vi "SPD.Config Read Test03a DTvsInsens.vi"(8 "Error In":errorcluster, 11 "SPD.Stand Ctrl in":T2={"spdDeviceSession"={"spdRef"=0, "connected"=FALSE, "spdName"="", "specification"={"diod case"=enum."default", "type"=enum."Unknown", "frequency"=enum."Unknown"}, "hidSPD.Controller"={"TSet"=0.0, "HV_bias"=0.0, "DDS_stb_code"=0}, "hidSPD.Sturtup Values"={"TSet"=0.0, "HV_bias"=0.0, "DDS_stb_code"=0}}, "DevBSession"={"DevBRef"="", "connected"=FALSE}, "FreqCSession"={"FreqCRef"="", "timeout"=0.0, "Gate"=0.0, "connected"=FALSE}, "8164BSession"={"Connection ID"=refnum, "Connected"=FALSE, "Info"="", "Slots Info"=[]}, "LeCroySession"={"LeCroySession"="", "connected"=FALSE}, "Events"={"DCRTest"=refnum, "Stop"=refnum}, "configFile"={"configFile ref"=refnum, "configFile path"=path "", "equipmentFile ref"=refnum}, "SPD.Meas Grid"={"DateTime"="", "DT"=[], "Insensitivity"=[], "Temprature"=[], "Stb_code"=[], "HV_Bias"=[]}, "SPD.Queues"={"state queue"=refnum}, "Console"=refnum} {"spdDeviceSession"."hidSPD.Sturtup Values"."HV_bias" format="%#_6p, V"; "spdDeviceSession"."hidSPD.Sturtup Values"."TSet" format="%#_6p, DegC"; "spdDeviceSession"."hidSPD.Controller"."HV_bias" format="%#_6p, V"; "spdDeviceSession"."hidSPD.Controller"."TSet" format="%#_6p, DegC"}) -> (0 "Error Out":errorcluster, 2 "DTvsInsens Params":T1, 3 "SPD.Stand Ctrl out":T2={"spdDeviceSession"={"spdRef"=0, "connected"=FALSE, "spdName"="", "specification"={"diod case"=enum."default", "type"=enum."Unknown", "frequency"=enum."Unknown"}, "hidSPD.Controller"={"TSet"=0.0, "HV_bias"=0.0, "DDS_stb_code"=0}, "hidSPD.Sturtup Values"={"TSet"=0.0, "HV_bias"=0.0, "DDS_stb_code"=0}}, "DevBSession"={"DevBRef"="", "connected"=FALSE}, "FreqCSession"={"FreqCRef"="", "timeout"=0.0, "Gate"=0.0, "connected"=FALSE}, "8164BSession"={"Connection ID"=refnum, "Connected"=FALSE, "Info"="", "Slots Info"=[]}, "LeCroySession"={"LeCroySession"="", "connected"=FALSE}, "Events"={"DCRTest"=refnum, "Stop"=refnum}, "configFile"={"configFile ref"=refnum, "configFile path"=path "", "equipmentFile ref"=refnum}, "SPD.Meas Grid"={"DateTime"="", "DT"=[], "Insensitivity"=[], "Temprature"=[], "Stb_code"=[], "HV_Bias"=[]}, "SPD.Queues"={"state queue"=refnum}, "Console"=refnum} {"spdDeviceSession"."hidSPD.Sturtup Values"."HV_bias" format="%#_6p, V"; "spdDeviceSession"."hidSPD.Sturtup Values"."TSet" format="%#_6p, DegC"; "spdDeviceSession"."hidSPD.Controller"."HV_bias" format="%#_6p, V"; "spdDeviceSession"."hidSPD.Controller"."TSet" format="%#_6p, DegC"})   [LabVIEW 2018]
uses:
  typedefs/SPD.Stand Ctrl.ctl
  Instruments/SPD HID Interface/hidSPDLibForLabView/LibVIs/hidSPD Controls/hidSPD Device Session.ctl
  Instruments/SPD HID Interface/hidSPDLibForLabView/LibVIs/hidSPD Controls/hidSPD.SPD specification.ctl
  Instruments/SPD HID Interface/hidSPDLibForLabView/LibVIs/hidSPD Controls/hidSPD SPD Diod Case.ctl
  Instruments/SPD HID Interface/hidSPDLibForLabView/LibVIs/hidSPD Controls/hidSPD SPD Type.ctl
  Instruments/SPD HID Interface/hidSPDLibForLabView/LibVIs/hidSPD Controls/hidSPD.STB Frequency.ctl
  Instruments/SPD HID Interface/hidSPDLibForLabView/LibVIs/hidSPD Controls/hidSPD Controller.ctl
  Instruments/KC705 DevBoard/typedefs/DevB.Session.ctl
  Instruments/KeySight 53230A/typedefs/FreqC.Session.ctl
  Instruments/KeySight 8164B/KeySight 8164B LAN InstrLib/typedefs/KeySight 8164B control.ctl
  Instruments/LeCroy SDA830/typedefs/LeCroy.Session.ctl
  typedefs/SPD.Events.ctl
  SPD.Config File ctrl.ctl
  <vilib>/Utility/config.llb/Config Data RefNum.ctl
  typedefs/SPD.Meas Grid.ctl
  typedefs/SPD.Queues.ctl
  typedefs/SPD.Stand state.ctl
  SPD Measurements/DT&Insensitivity/typedefs/SPD.DT&Insens Test Params.ctl
  <vilib>/Utility/config.llb/Read Key (I32).vi
  <vilib>/Utility/config.llb/Read Key (Double).vi
  <vilib>/Utility/config.llb/Read Key (String).vi
  <vilib>/Utility/config.llb/NI_LVConfig.lvlib
  Instruments/KeySight 8164B/KeySight 8164B LAN InstrLib.lvlib
  Instruments/SPD HID Interface/hidSPDLibForLabView/hidSPDLibForLabView.lvlib
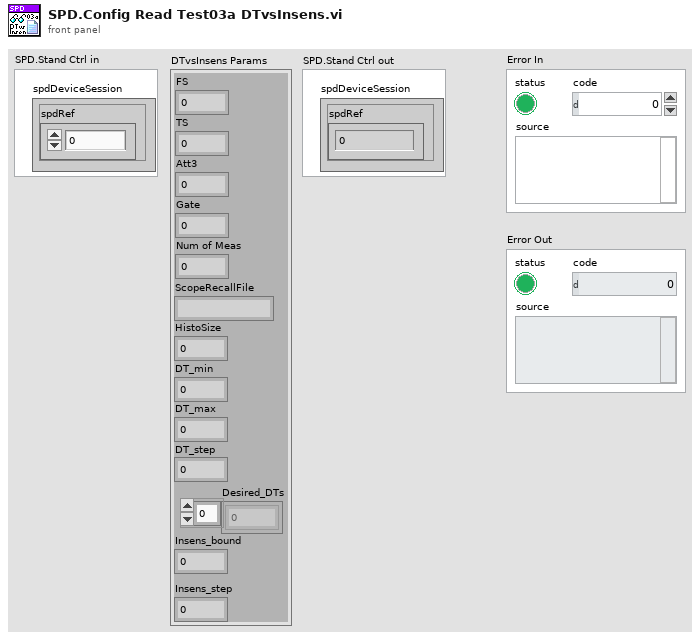
[diagram p1: front panel]
types:
  T1 = typedef "SPD.DT&Insens Test Params.ctl" = cluster{"FS":i32, "TS":i32, "Att3":dbl, "Gate":dbl, "Num of Meas":i32, "ScopeRecallFile":string, "HistoSize":i32, "DT_min":u16, "DT_max":u16, "DT_step":u16, "Desired_DTs":dbl[], "Insens_bound":u16, "Insens_step":u16}
  T2 = typedef "SPD.Stand Ctrl.ctl" = cluster{"spdDeviceSession":T3, "DevBSession":T9, "FreqCSession":T10, "8164BSession":T11, "LeCroySession":T12, "Events":T13, "configFile":T14, "SPD.Meas Grid":T16, "SPD.Queues":T17, "Console":refnum<vi>}
  T3 = typedef "hidSPDLibForLabView.lvlib/hidSPD Device Session.ctl" = cluster{"spdRef":u64, "connected":bool, "spdName":string, "specification":T4, "hidSPD.Controller":T8, "hidSPD.Sturtup Values":T8}
  T4 = typedef "hidSPDLibForLabView.lvlib/hidSPD.SPD specification.ctl" = cluster{"diod case":T5, "type":T6, "frequency":T7}
  T5 = typedef "hidSPDLibForLabView.lvlib/hidSPD SPD Diod Case.ctl" = enum16{"Unknown", "default", "butterfly"}
  T6 = typedef "hidSPDLibForLabView.lvlib/hidSPD SPD Type.ctl" = enum16{"Unknown", "Free Run", "Gate"}
  T7 = typedef "hidSPDLibForLabView.lvlib/hidSPD.STB Frequency.ctl" = enum16{"Unknown", "312", "1250"}
  T8 = typedef "hidSPDLibForLabView.lvlib/hidSPD Controller.ctl" = cluster{"TSet":sgl, "HV_bias":sgl, "DDS_stb_code":u16}
  T9 = typedef "DevB.Session.ctl" = cluster{"DevBRef":refnum<visa-resource-name>, "connected":bool}
  T10 = typedef "FreqC.Session.ctl" = cluster{"FreqCRef":refnum<visa-resource-name>, "timeout":dbl, "Gate":dbl, "connected":bool}
  T11 = typedef "KeySight 8164B LAN InstrLib.lvlib/KeySight 8164B control.ctl" = cluster{"Connection ID":refnum<k5>, "Connected":bool, "Info":string, "Slots Info":string[]}
  T12 = typedef "LeCroy.Session.ctl" = cluster{"LeCroySession":refnum<visa-resource-name>, "connected":bool}
  T13 = typedef "SPD.Events.ctl" = cluster{"DCRTest":refnum<user-event>, "Stop":refnum<user-event>}
  T14 = typedef "SPD.Config File ctrl.ctl" = cluster{"configFile ref":T15, "configFile path":path, "equipmentFile ref":T15}
  T15 = typedef "NI_LVConfig.lvlib/Config Data RefNum.ctl" = refnum<k1>
  T16 = typedef "SPD.Meas Grid.ctl" = cluster{"DateTime":string, "DT":dbl[], "Insensitivity":dbl[], "Temprature":dbl[], "Stb_code":dbl[], "HV_Bias":dbl[][][][]}
  T17 = typedef "SPD.Queues.ctl" = cluster{"state queue":refnum<queue>}
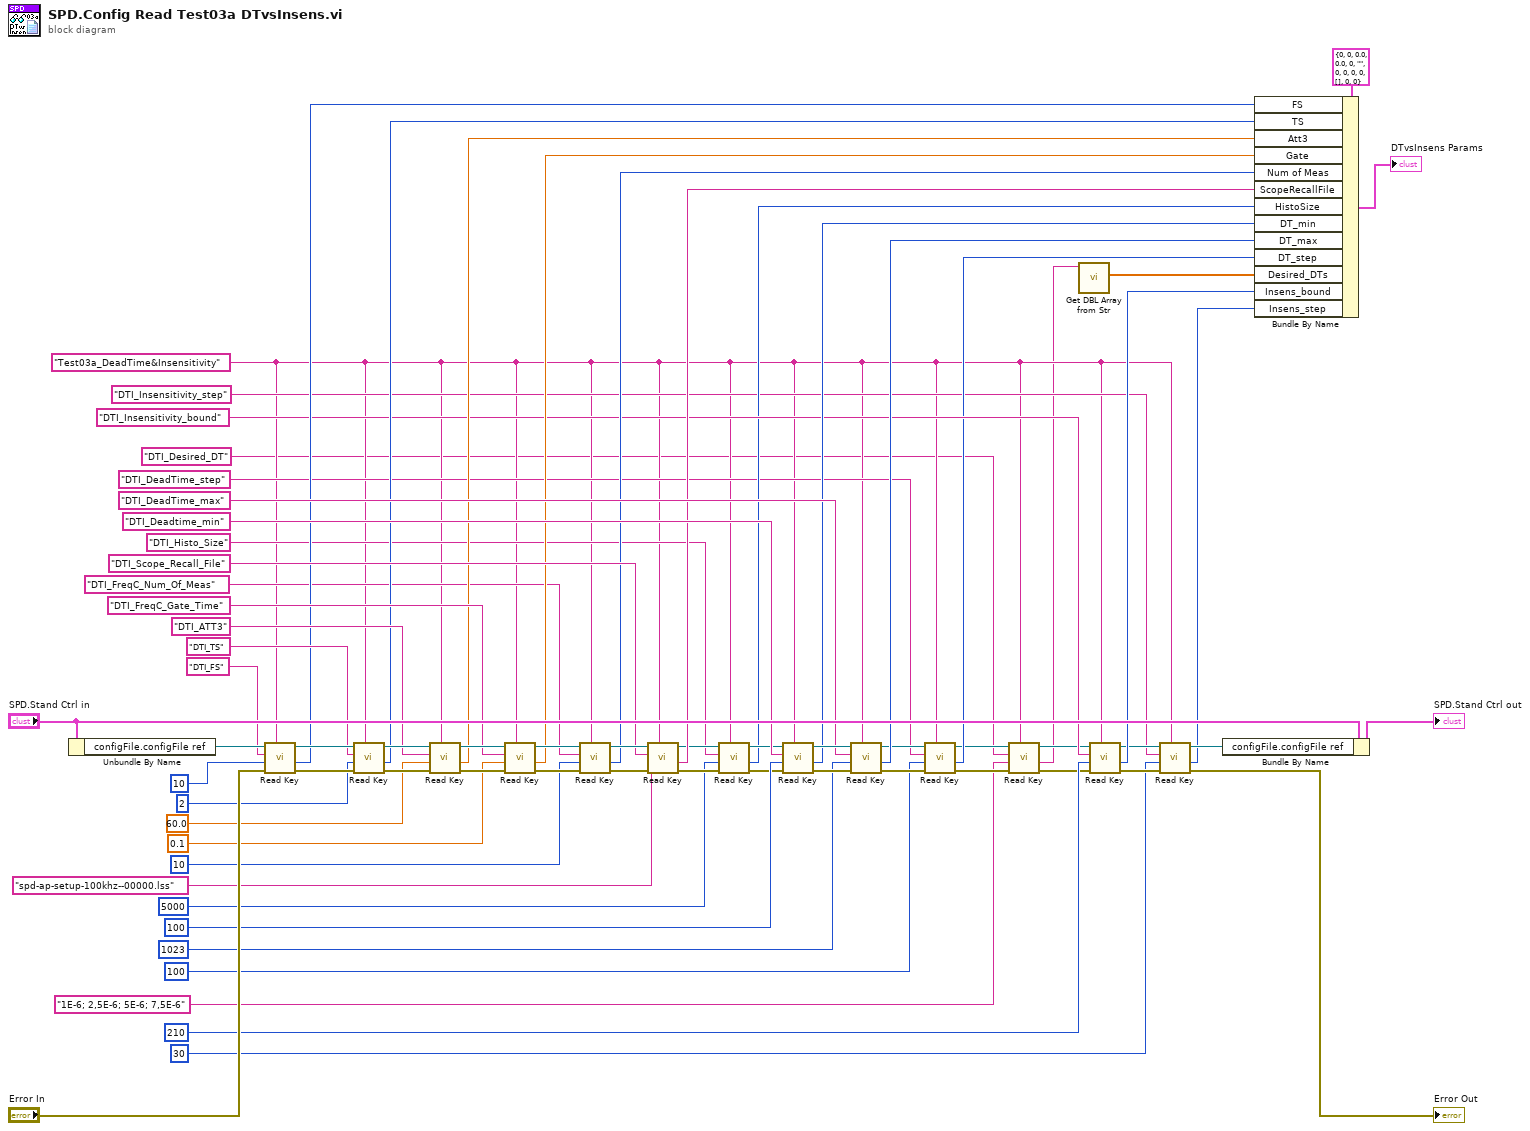
[diagram p0: block diagram]
diagram:
  w5 = "Test03a_DeadTime&Insensitivity" ("section")
  n1 = Unbundle By Name("SPD.Stand Ctrl in") -> ("configFile.configFile ref"=w71:T15)
  n2 = call-poly <vilib>:"Read Key.vi"("section"=w5, "error in (no error)"="Error In", "default value"=10, "key"="DTI_FS", "refnum"=w71) -> ("error out"=w67:errorcluster, "value"=w43:i32, "refnum out"=w66:T15)  [unwired: 3 in, 1 out]
  n3 = call-poly <vilib>:"Read Key.vi"("section"=w5, "error in (no error)"=w67, "default value"=2, "key"="DTI_TS", "refnum"=w66) -> ("error out"=w62:errorcluster, "value"=w42:i32, "refnum out"=w63:T15)  [unwired: 3 in, 1 out]
  n4 = call-poly <vilib>:"Read Key.vi"("section"=w5, "error in (no error)"=w62, "default value"=60.0, "key"="DTI_ATT3", "refnum"=w63) -> ("error out"=w58:errorcluster, "value"=w41:dbl, "refnum out"=w59:T15)  [unwired: 3 in, 1 out]
  n5 = call-poly <vilib>:"Read Key.vi"("section"=w5, "error in (no error)"=w58, "default value"=0.1, "key"="DTI_FreqC_Gate_Time", "refnum"=w59) -> ("error out"=w54:errorcluster, "value"=w40:dbl, "refnum out"=w55:T15)  [unwired: 3 in, 1 out]
  n6 = call-poly <vilib>:"Read Key.vi"("section"=w5, "error in (no error)"=w54, "default value"=10, "key"="DTI_FreqC_Num_Of_Meas", "refnum"=w55) -> ("error out"=w50:errorcluster, "value"=w39:i32, "refnum out"=w52:T15)  [unwired: 3 in, 1 out]
  n7 = call-poly <vilib>:"Read Key.vi"("section"=w5, "error in (no error)"=w50, "default value"="spd-ap-setup-100khz--00000.lss" ("key"), "key"="DTI_Scope_Recall_File", "refnum"=w52) -> ("error out"=w28:errorcluster, "value"=w38:string, "refnum out"=w29:T15)  [unwired: 3 in, 1 out]
  n8 = call-poly <vilib>:"Read Key.vi"("section"=w5, "error in (no error)"=w28, "default value"=5000, "key"="DTI_Histo_Size", "refnum"=w29) -> ("error out"=w27:errorcluster, "value"=w25:i32, "refnum out"=w26:T15)  [unwired: 3 in, 1 out]
  n9 = call-poly <vilib>:"Read Key.vi"("section"=w5, "error in (no error)"=w27, "default value"=100, "key"="DTI_Deadtime_min", "refnum"=w26) -> ("error out"=w48:errorcluster, "value"=w37:i32, "refnum out"=w49:T15)  [unwired: 3 in, 1 out]
  n10 = call-poly <vilib>:"Read Key.vi"("section"=w5, "error in (no error)"=w48, "default value"=1023, "key"="DTI_DeadTime_max", "refnum"=w49) -> ("error out"=w21:errorcluster, "value"=w36:i32, "refnum out"=w22:T15)  [unwired: 3 in, 1 out]
  n11 = call-poly <vilib>:"Read Key.vi"("section"=w5, "error in (no error)"=w21, "default value"=100, "key"="DTI_DeadTime_step", "refnum"=w22) -> ("error out"=w7:errorcluster, "value"=w18:i32, "refnum out"=w9:T15)  [unwired: 3 in, 1 out]
  n12 = call-poly <vilib>:"Read Key.vi"("section"=w5, "error in (no error)"=w7, "default value"="1E-6; 2,5E-6; 5E-6; 7,5E-6" ("key"), "key"="DTI_Desired_DT", "refnum"=w9) -> ("error out"=w6:errorcluster, "value"=w2:string, "refnum out"=w8:T15)  [unwired: 3 in, 1 out]
  n13 = call "Get DBL Array from Str.vi"("String"=w2) -> ("Array"=w1:dbl[])  [unwired: 10 in]
  n14 = call-poly <vilib>:"Read Key.vi"("section"=w5, "error in (no error)"=w6, "default value"=210, "key"="DTI_Insensitivity_bound", "refnum"=w8) -> ("error out"=w14:errorcluster, "value"=w32:i32, "refnum out"=w16:T15)  [unwired: 3 in, 1 out]
  n15 = call-poly <vilib>:"Read Key.vi"("section"=w5, "error in (no error)"=w14, "default value"=30, "key"="DTI_Insensitivity_step", "refnum"=w16) -> ("error out"=→"Error Out":errorcluster, "value"=w10:i32, "refnum out"=w15:T15)  [unwired: 3 in, 1 out]
  n16 = Bundle By Name(cluster="SPD.Stand Ctrl in", "configFile.configFile ref"=w15) -> (→"SPD.Stand Ctrl out":T2)
  n17 = Bundle By Name(cluster=T1 {"FS"=0, "TS"=0, "Att3"=0.0, "Gate"=0.0, "Num of Meas"=0, "ScopeRecallFile"="", "HistoSize"=0, "DT_min"=0, "DT_max"=0, "DT_step"=0, "Desired_DTs"=[], "Insens_bound"=0, "Insens_step"=0} ("DTvsInsens Params"), "FS"=w43, "TS"=w42, "Att3"=w41, "Gate"=w40, "Num of Meas"=w39, "ScopeRecallFile"=w38, "HistoSize"=w25, "DT_min"=w37, "DT_max"=w36, "DT_step"=w18, "Desired_DTs"=w1, "Insens_bound"=w32, "Insens_step"=w10) -> (→"DTvsInsens Params":T1)
